vi "Initialize.vi"(8 "error in (no error)":errorcluster, 9 "Reset (True)":bool=TRUE, 10 "ID Query (True)":bool=TRUE, 11 "VISA resource name":refnum<visa-resource-name>) -> (0 "error out":errorcluster, 2 "idn string":string, 3 "VISA resource name out":refnum<visa-resource-name>)   [LabVIEW 2018, in "Counter.lvlib" / "PICOTEST U62XXA series.lvlib"]
doc: "Establishes communication with the instrument and optionally performs an instrument identification query and/or an instrument reset. It also places the instrument in a default state needed for other instrument driver operations. Therefore, call this VI before calling other instrument driver VIs for this instrument. Generally, you need to call the Initialize VI only once at the beginning of an application."
uses:
  PICOTEST U62XXA series.lvlib
panel:
  # "(c) 2009 PICOTEST CORP.  ALL RIGHTS RESERVED."
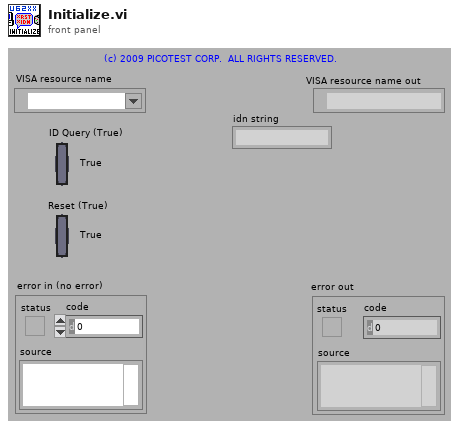
[diagram p1: front panel]
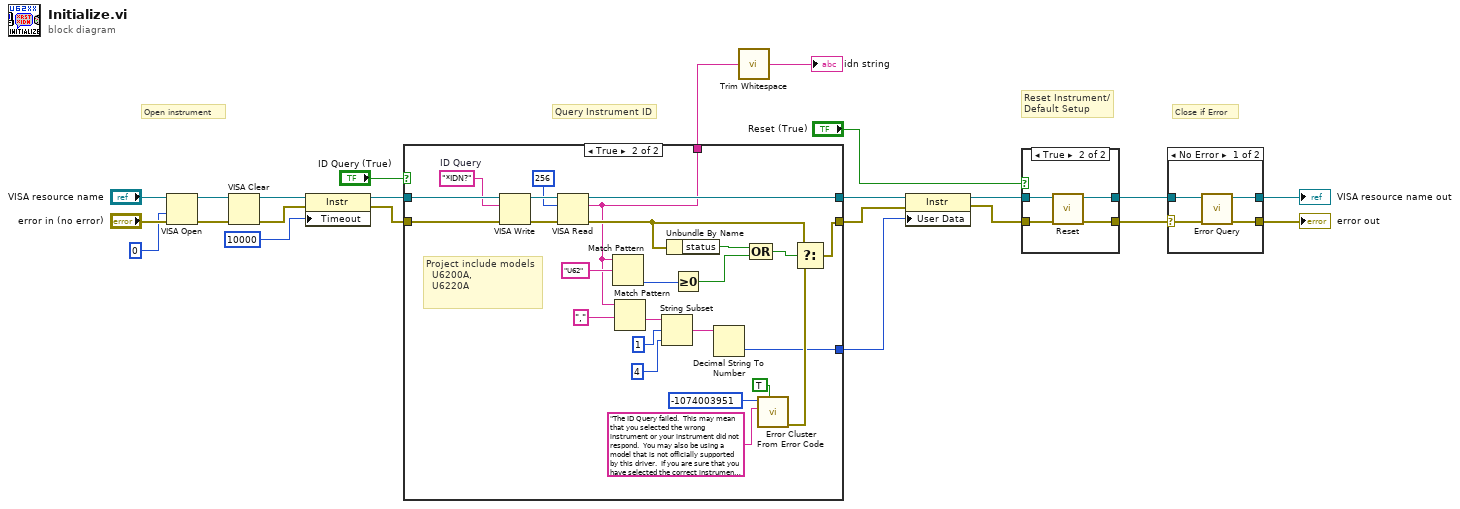
[diagram p0: block diagram]
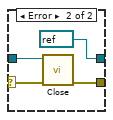
[diagram p2: hidden frame]
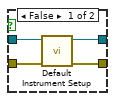
[diagram p3: hidden frame]
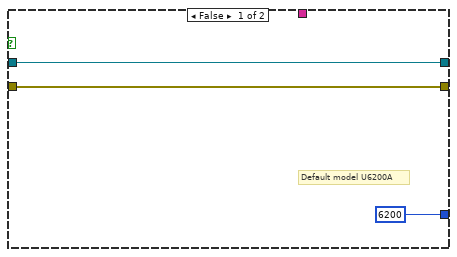
[diagram p4: hidden frame]
diagram:
  # "Close if Error"
  # "Query Instrument ID"
  # "Reset Instrument/\nDefault Setup"
  # "Open instrument"
  n1 = VISA Open(access mode=u32 0, error in (no error)="error in (no error)", VISA resource name="VISA resource name") -> (VISA resource name=w16:refnum<visa-resource-name>, error out=w15:errorcluster)  [unwired: 2 in]
  n2 = VISA Clear(VISA resource name=w16, error in (no error)=w15) -> (VISA resource name out=w14:refnum<visa-resource-name>, error out=w13:errorcluster)
  n3 = property class="Instr"(reference=w14, error in=w13, "Timeout"=u32 10000 ("General Settings:Timeout Value")) -> (reference out=w19:refnum<visa-resource-name>, error out=w18:errorcluster)
  n4 = case shown="True" "ID Query (True)" {
    tunnel: [w25 w51] -> w5
    tunnel: [w26 w48] -> w7
    tunnel: w19 -> [w26 w49]
    tunnel: w18 -> [w25 w50]
    tunnel: [6200 w29] -> w3
    tunnel: [_ w27] -> w2
    frame False {
      # "Default model U6200A"
    }
    frame True {
      w43 = "*IDN?"  # ID Query
      # "Project include models\n  U6200A,\n  U6220A"
      n5 = VISA Write(VISA resource name=w49, write buffer=w43, error in (no error)=w50) -> (VISA resource name out=w47:refnum<visa-resource-name>, error out=w46:errorcluster)  [unwired: 1 out]
      n6 = VISA Read(VISA resource name=w47, byte count=u32 256, error in (no error)=w46) -> (VISA resource name out=w48:refnum<visa-resource-name>, read buffer=w27:string, error out=w37:errorcluster)  [unwired: 1 out]
      n7 = Match Pattern(string=w27, regular expression="U62") -> (offset past match=w38:i32)  [unwired: 1 in, 3 out]
      n8 = Match Pattern(string=w27, regular expression=",") -> (after substring=w32:string)  [unwired: 1 in, 3 out]
      n9 = String Subset(string=w32, offset (0)=1, length (rest)=4 ("length (rest)")) -> (substring=w31:string)
      n10 = Unbundle By Name(w37) -> ("status"=w36:bool)
      n11 = Greater Or Equal To 0?(x=w38) -> (x >= 0?=w35:bool)
      n12 = Decimal String To Number(string=w31) -> (number=w29:i32)  [unwired: 2 in, 1 out]
      n13 = Compound Arithmetic op=OR(w36, w35) -> (w34:bool)
      n14 = call <vilib>:"Error Cluster From Error Code.vi"("show call chain? (False)"=TRUE, "error message (\"\")"="The ID Query failed.  This may mean that you selected the wrong instrument or your instrument did not respond.  You may also be using a model that is not officially supported by this driver.  If you are sure that you have selected the correct instrument and it is responding, try disabling the ID Query." ("Source (VI Name)"), "error code (0)"=-1074003951 ("Code")) -> ("error out"=w42:errorcluster)  [unwired: 6 in]
      n15 = Select(t=w37, s=w34, f=w42) -> (s? t:f=w51:errorcluster)
    }
  }
  n16 = call <vilib>:"Trim Whitespace.vi"("string"=w2) -> ("trimmed string"=→"idn string":string)  [unwired: 1 in]
  n17 = property class="Instr"(reference=w7, error in=w5, "User Data"=w3) -> (reference out=w6:refnum<visa-resource-name>, error out=w4:errorcluster)
  n18 = case shown="True" "Reset (True)" {
    tunnel: w4 -> [w55 w57]
    tunnel: [w54 w59] -> w9
    tunnel: [w53 w58] -> w10
    tunnel: w6 -> [w52 w56]
    frame False {
      n19 = call "Default Instrument Setup.vi"("error in (no error)"=w55, "VISA resource name"=w52) -> ("error out"=w54:errorcluster, "VISA resource name out"=w53:refnum<visa-resource-name>)  [unwired: 8 in]
    }
    frame True {
      n20 = call "Reset.vi"("error in (no error)"=w57, "VISA resource name"=w56) -> ("error out"=w59:errorcluster, "VISA resource name out"=w58:refnum<visa-resource-name>)  [unwired: 8 in]
    }
  }
  n21 = case shown="No Error" w9 {
    selector: w9 -> [w61 w65]
    tunnel: w10 -> [w60 w66]
    tunnel: [w63 refnum<visa-resource-name> refnum ("VISA resource name out")] -> w12
    tunnel: [w62 w67] -> w11
    frame No Error {
      n22 = call "Error Query.vi"("error in (no error)"=w61, "VISA resource name"=w60) -> ("error out"=w62:errorcluster, "VISA resource name out"=w63:refnum<visa-resource-name>)  [unwired: 6 in, 2 out]
    }
    frame Error {
      n23 = call "Close.vi"("error in (no error)"=w65, "VISA resource name"=w66) -> ("error out"=w67:errorcluster)  [unwired: 9 in]
    }
  }
  "VISA resource name out" <- w12
  "error out" <- w11
